vi "Write (I16 Data Ref).vi"(0 "disk streaming in":refnum<class "Disk Streaming.lvclass">, 1 "sample data":refnum<data-value>, 2 "elements in region":u32, 3 "elements remaining":u32, 5 "error in (no error)":errorcluster) -> (13 "finished":bool, 14 "disk streaming out":refnum<class "Disk Streaming.lvclass">, 18 "number of pending writes":u32, 19 "error out":errorcluster)   [LabVIEW 2021, in "Disk Streaming.lvclass"]
doc: "Writes data to a file in the streaming process controlled by a disk streaming instance and generates status information. For more information about the disk streaming instance refer to the <B>Open.vi</B> context help.\n\nUse this VI when streaming to disk using the TDMS Advanced Data Reference I/O functions (the disk streaming instance was created by the <B>Open.vi</B> with the <B>disk read (F) / write (T)</B> input set to true and the <B>I/O mode</B> input set to \"Data Reference\"). The streaming process requires the execution of the following sequence in a loop:\n1. Use the <B>Get Next Transfer Size.vi</B> to obtain the number of elements to transfer in the current iteration. If this VI returns zero, then the streaming is complete.\n2. Call the Acquire Read Region FIFO method on the Target to Host FIFO transferring the data from the FPGA Target to acquire the buffer to write to the file. Use the value returned by the <B>Get Next Transfer Size.vi</B> on the \"Number of Elements\" input of the FIFO method.\n3. Call this VI using the outputs returned by the FIFO method.\n\nInputs:\n\n<B>disk streaming in</B>: Disk streaming instance input.\n\n<B>sample data</B>: External Data Value Reference (EDVR) referencing the array of I16s to write to the file. Wire the \"Read Region Reference\" output of the FIFO method acquiring the Target to Host FIFO buffer to write to the file to this input.\n\n<B>elements in region</B>: The size of the array of I16s referenced by the EDVR passed on the <B>sample data</B> input. Wire the \"Elements In Region\" output of the FIFO method acquiring the Target to Host FIFO buffer to write to the file to this input.\n\n<B>elements remaining</B>: Set this input to the number of additional elements remaining in the host DMA buffer that are available for reading. This input is used only in the calculation of the Host DMA buffer utilization status. Wire the \"Elements Remaining\" output of the FIFO method acquiring the Target to Host FIFO buffer to write to the file to this input.\n\nOutputs:\n\n<B>disk streaming out</B>: Disk streaming instance output. Pass this output to the other Disk Streaming VIs to perform the streaming.\n\n<B>number of pending writes</B>: The number of asynchronous writes that are currently running in the background. Use the <B>Get Status.vi</B> to obtain additional status information.\n\n<B>finished</B>: Indicates whether the streaming is finished."
uses:
  Disk Streaming.lvclass
  Disk Streaming.lvclass/Disk Streaming.ctl
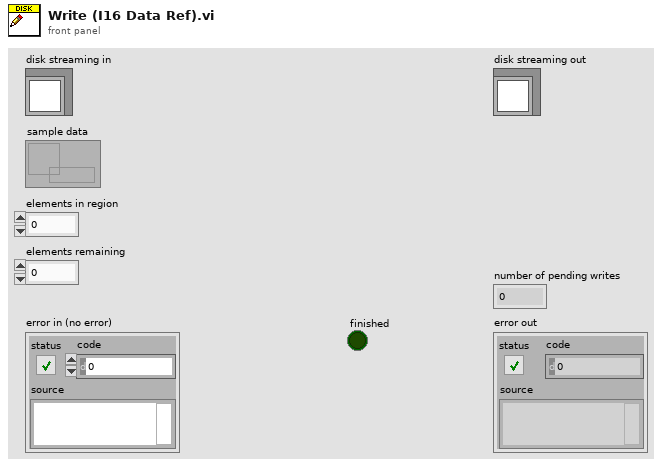
[diagram p1: front panel]
types:
  T1 = typedef "Disk Streaming.lvclass/Data.ctl" = cluster{"tdms file":refnum<k34>, "group name":string, "channel name":string, "max operations":u32, "timeout (s)":dbl, "data type size (bytes)":u64, "writing":bool, "I/O mode":T2, "# of blocks":u32, "block size divisor (bytes)":u32, "file position (elements)":u64, "file size (elements)":i64, "file size (samples)":i64, "block size (elements)":u64, "block size (samples)":u64, "quantum size (elements)":u64, "quantum size (samples)":u64, "samples remaining":i64, "elements transferred":u64, "finished":bool, "preview size":i32, "preview quantum size (elements)":u64, "preview quantum size (samples)":u64, "DMA buffer size (elements)":u32, "pending block sizes (bytes)":u64[]}
  T2 = typedef "Disk Streaming.lvclass/IO mode.ctl" = enum16{"Synchronous", "Asynchronous", "Data Reference"}
  T3 = typedef "Disk Streaming.lvclass/Status.ctl" = cluster{"finished":bool, "Host DMA buffer size (bytes)":u64, "Host DMA buffer utilization (bytes)":u64, "Disk maximum async operations":u32, "Disk pending async operations":u32, "preview data":i16[]}
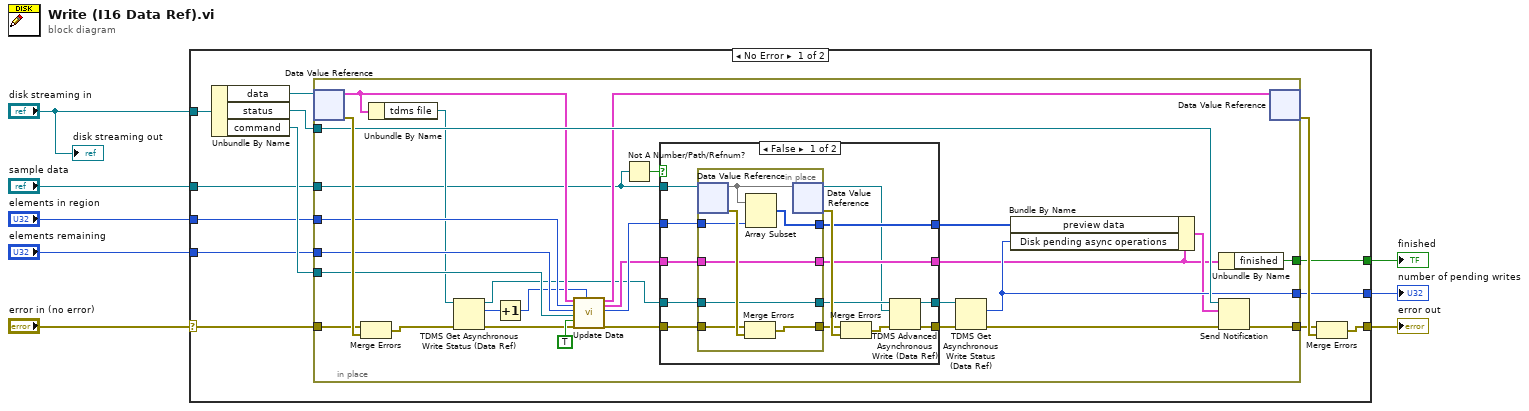
[diagram p0: block diagram]
diagram:
  n1 = case shown="No Error" "error in (no error)" {
    selector: "error in (no error)" -> [w19 w76]
    tunnel: [w18 w76] -> w7
    tunnel: "sample data" -> [w13 _]
    tunnel: [w16 _] -> w6
    tunnel: "elements remaining" -> [w12 _]
    tunnel: "disk streaming in" -> [w15 _]
    tunnel: [w10 _] -> w3
    tunnel: "elements in region" -> [w9 _]
    frame No Error {
      n2 = Unbundle By Name(w15) -> ("data"=w14:refnum<data-value>, "status"=w11:refnum<notifier>, "command"=w21:refnum<notifier>)
      n3 = in-place {
        in-place-border: w19 -> [w47]
        in-place-border: [w37] -> w17
        in-place-border: [w44] -> w16
        in-place-border: w21 -> [w40]
        in-place-border: w13 -> [w22]
        in-place-border: w12 -> [w41]
        in-place-border: w11 -> [w48]
        in-place-border: [w36] -> w10
        in-place-border: w9 -> [w35]
        n4 = in-place-dvr #1(w14) -> (w29:T1, w49:errorcluster)
        n5 = Merge Errors(w47, w49) -> (w28:errorcluster)
        n6 = Unbundle By Name(w29) -> ("tdms file"=w27:refnum<k34>)
        n7 = TDMS Get Asynchronous Write Status (Data Ref)(8:w28, 11:w27) -> (0:w26:errorcluster, 2:w24:u32, 3:w25:refnum<k34>)
        n8 = Increment(x=w24) -> (x+1=w23:u32)
        n9 = call "Update Data.vi"("data in"=w29, "block size (elements)"=w35, "(empty) elements remaining"=w41, "command"=w40, "writing?"=TRUE, "error in (no error)"=w26, "pending blocks in host buffer"=w23) -> ("data out"=w42:T1, "status"=w31:T3, "preview size (elements)"=w50:i32, "error out"=w34:errorcluster)  [unwired: 7 in, 2 out]
        n10 = Not A Number/Path/Refnum?(number/path/refnum=w22) -> (NaN/Path/Refnum?=w32:bool)
        n11 = case shown="False" w32 {
          tunnel: [w63 w73] -> w46
          tunnel: [w62 w74] -> w45
          tunnel: w34 -> [w61 w73]
          tunnel: w31 -> [w60 w75]
          tunnel: w25 -> [w59 w74]
          tunnel: [w52 w75] -> w30
          tunnel: w50 -> [w57 _]
          tunnel: [w56 _] -> w33
          tunnel: w22 -> [w53 _]
          frame False {
            n12 = in-place {
              in-place-border: w61 -> [w67]
              in-place-border: w60 -> [w65]
              in-place-border: w59 -> [w71]
              in-place-border: [w65] -> w52
              in-place-border: [w71] -> w58
              in-place-border: w57 -> [w69]
              in-place-border: [w68] -> w56
              in-place-border: [w66] -> w55
              n13 = in-place-dvr #2(w53) -> (w70:i16[], w72:errorcluster)
              n14 = Merge Errors(w67, w72) -> (w66:errorcluster)
              n15 = Array Subset(array=w70, length=w69) -> (w68:i16[])  [unwired: 1 in]
              n16 = in-place-dvr #2(w70) -> (w51:refnum<data-value>, w64:errorcluster)
            }
            n17 = Merge Errors(w55, w64) -> (w54:errorcluster)
            n18 = TDMS Advanced Asynchronous Write (Data Ref)(8:w54, 10:w51, 11:w58) -> (0:w63:errorcluster, 3:w62:refnum<k34>)  [unwired: 1 in]
          }
          frame True {
          }
        }
        n19 = TDMS Get Asynchronous Write Status (Data Ref)(8:w46, 11:w45) -> (0:w38:errorcluster, 2:w44:u32)  [unwired: 1 out]
        n20 = Bundle By Name(cluster=w30, "preview data"=w33, "Disk pending async operations"=w44) -> (w43:T3)
        n21 = Unbundle By Name(w30) -> ("finished"=w36:bool)
        n22 = Send Notification(notification=w43, notifier=w48, error in (no error)=w38) -> (error out=w37:errorcluster)  [unwired: 1 out]
        n23 = in-place-dvr #1(w42) -> (w20:errorcluster)  [unwired: 1 out]
      }
      n24 = Merge Errors(w17, w20) -> (w18:errorcluster)
    }
    frame Error {
    }
  }
  "error out" <- w7
  "number of pending writes" <- w6
  "finished" <- w3
  "disk streaming out" <- "disk streaming in"
